vi "FPGA Target 2.vi"() -> ()   [LabVIEW 2025]
uses:
  <vilib>/Platform/TimedLoop/XDataNode/wakeup.ctl
  <vilib>/Platform/TimedLoop/XDataNode/XDNodeRunTimeDep.lvlib
  <vilib>/Platform/TimedLoop/XDataNode/nitl_modes.ctl
  <vilib>/Platform/TimedLoop/XDataNode/timing_clust.ctl
  <vilib>/Platform/TimedLoop/XDataNode/XDataNode.xnode
  <vilib>/rvi/DataTransferAndStorage/Container/XNode/niFpgaContainer.xnode
  Templates/FPGA Wizard Templates.lvlib
  <vilib>/rvi/interface/RandomDataEmulation/nirviRandomDataFpgaReadWriteTemplate.vi
panel:
  out "Actual Analog Input Loop Period (usec)":u32
  out "Actual Analog Output Loop Period (usec)":u32
  out "Actual Digital Loop Period (usec)":u32
  out "Actual DMA Loop Period (usec)":u32
  in  "Analog Input Loop Timer (uSec)":u32=10
  in  "Digital Loop Timer (uSec)":u32=10
  in  "Analog Output Loop Timer (uSec)":u32=10
  in  "DMA.Enable":bool
  in  "DMA.MinimumSamples":u32=100000 caption="DMA Loop Timer (uSec)"
  out "DMA.Timeout":bool
  in  "DMA.Timeout.Reset":bool
  in  "DMA Loop Timer (uSec)":u32=10
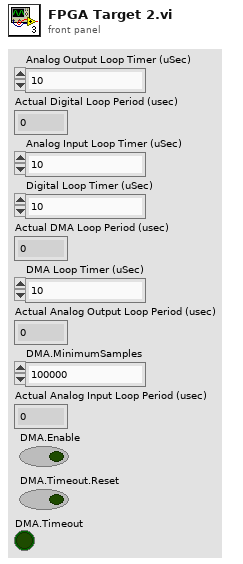
[diagram p1: front panel]
types:
  T1 = typedef "XDNodeRunTimeDep.lvlib/timing_clust.ctl" = cluster{"Expected End [f-1]":u64, "Actual End [f-1]":u64, "Finished Late? [f-1]":bool, "Expected End [i-1]":u64, "Actual End [i-1]":u64, "Finished Late? [i-1]":bool, "Expected Start [i]":u64, "Actual Start [i]":u64, "Expected Start [f]":u64, "Actual Start [f]":u64, "Source Name":string, "Structure Name":string, "Period":i64, "Deadline":i64, "Offset":i64, "Start":i64, "Priority":i32, "Timeout":i32, "Mode":T2, "Wakeup Reason":T3, "Error":errorcluster, "Source Type":string, "Secondary Source Type":string, "Global End Time":u64, "Global Start Time":u64, "Frame Duration":u64, "Iteration Duration":u64, "Assigned CPU":i32, "I/O Scan Engine Mode":u32}
  T2 = typedef "XDNodeRunTimeDep.lvlib/nitl_modes.ctl" = enum32{"No Change", "Process missed periods, maintain original phase", "Discard missed periods, maintain original phase", "Process missed periods, ignore original phase", "Discard missed periods, ignore original phase"}
  T3 = typedef "XDNodeRunTimeDep.lvlib/wakeup.ctl" = enum32{"Normal", "Aborted", "Asynchronous wakeup", "Timing source error", "Timed loop error", "Timeout"}
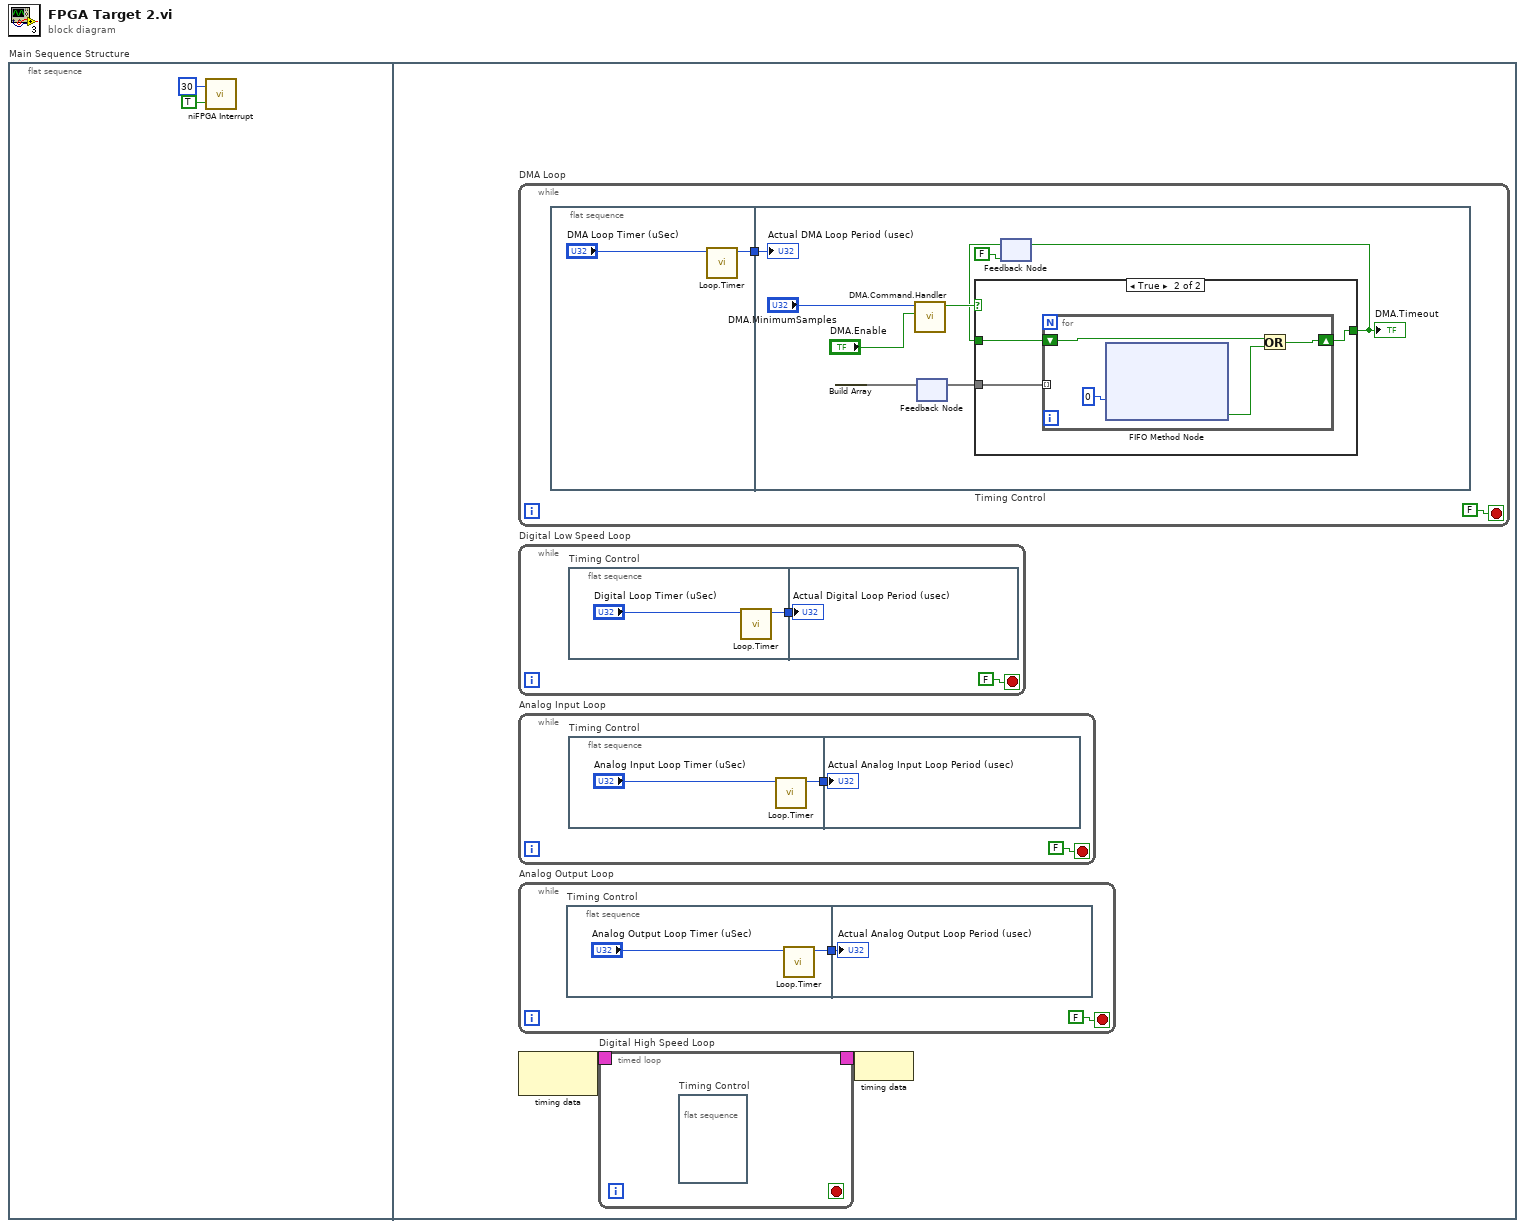
[diagram p0: block diagram]
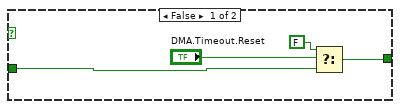
[diagram p2: hidden frame]
diagram:
  n1 = flat-sequence "Main Sequence Structure" {
    frame #0 {
      n2 = call <vilib>:"niFPGA Interrupt.vi"("Wait Until Cleared (F)"=TRUE, "IRQ Number (0)"=u8 30) -> ()  [unwired: 1 in]
    }
    frame #1 {
      # "FPGA Addon Code"
      n3 = while "DMA Loop" {
        stop <- FALSE stop-if-true
        n4 = flat-sequence "Timing Control" {
          tunnel: [w11] -> w9
          tunnel: w9 -> [w13]
          frame #0 {
            n5 = call "Loop.Timer.vi"("Loop Timer (uSec)"="DMA Loop Timer (uSec)") -> ("Actual Loop Period (usec)"=w11:u32)  [unwired: 10 in]
          }
          frame #1 {
            n6 = Build Array "Build Array"() -> (w19:void[])  [unwired: 1 in]
            n7 = call "DMA.Command.Handler.vi"("DMA.Enable"="DMA.Enable", "DMA.MinimumSamples"="DMA.MinimumSamples") -> ("Transfer"=w15:bool)  [unwired: 9 in]
            n8 = feedback #1() -> (w18:void[])  [unwired: 1 in]
            n9 = feedback-in #1(w19) -> ()
            n10 = feedback #2(FALSE ("t")) -> (w14:bool)
            n11 = case shown="True" w15 {
              tunnel: w18 -> [_ w28]
              tunnel: w14 -> [w23 w27]
              tunnel: [w22 w26] -> w17
              frame False {
                n12 = Select(t=FALSE, s="DMA.Timeout.Reset", f=w23) -> (s? t:f=w22:bool)
              }
              frame True {
                n13 = for {
                  shift-right: [w30] -> w26
                  shift-left: w27 -> [w29]
                  tunnel: w28 -> [_] mode=indexing
                  n14 = xnode ("FIFO Method Node")("Timeout"=0) -> ("Timed Out?"=w31:bool)  [unwired: 2 in, 1 out]
                  n15 = Or(x=w29, y=w31) -> (x .or. y?=w30:bool)
                }
              }
            }
            "DMA.Timeout" <- w17
            n16 = feedback-in #2(w17) -> ()
            "Actual DMA Loop Period (usec)" <- w13
          }
        }
      }
      n17 = while "Digital Low Speed Loop" {
        stop <- FALSE stop-if-true
        n18 = flat-sequence "Timing Control" {
          tunnel: [w45] -> w43
          tunnel: w43 -> [w47]
          frame #0 {
            n19 = call "Loop.Timer.vi"("Loop Timer (uSec)"="Digital Loop Timer (uSec)") -> ("Actual Loop Period (usec)"=w45:u32)  [unwired: 10 in]
          }
          frame #1 {
            "Actual Digital Loop Period (usec)" <- w47
          }
        }
      }
      n20 = while "Analog Input Loop" {
        stop <- FALSE stop-if-true
        n21 = flat-sequence "Timing Control" {
          tunnel: [w40] -> w38
          tunnel: w38 -> [w42]
          frame #0 {
            n22 = call "Loop.Timer.vi"("Loop Timer (uSec)"="Analog Input Loop Timer (uSec)") -> ("Actual Loop Period (usec)"=w40:u32)  [unwired: 10 in]
          }
          frame #1 {
            "Actual Analog Input Loop Period (usec)" <- w42
          }
        }
      }
      n23 = while "Analog Output Loop" {
        stop <- FALSE stop-if-true
        n24 = flat-sequence "Timing Control" {
          tunnel: [w35] -> w33
          tunnel: w33 -> [w37]
          frame #0 {
            n25 = call "Loop.Timer.vi"("Loop Timer (uSec)"="Analog Output Loop Timer (uSec)") -> ("Actual Loop Period (usec)"=w35:u32)  [unwired: 10 in]
          }
          frame #1 {
            "Actual Analog Output Loop Period (usec)" <- w37
          }
        }
      }
      n26 = node-c288() -> (w4:T1)  [unwired: 1 in]
      n27 = timed-loop "Digital High Speed Loop" {
        timing: w4 -> [_]
        timing-out: [_] -> w3
        stop <- _ stop-if-true
        n28 = flat-sequence "Timing Control" {
          frame #0 {
          }
        }
      }
      n29 = node-c288 ("Output Node")(w3) -> ()
    }
  }
